vi "transfer char run_subvi_14_2014 05 29_JWb.vi"(0 "VISA session":refnum<visa-resource-name>="GPIB0::17::INSTR", 1 "Y2 axis settings":T6={"Y2 axis on/off"=FALSE, "MINIMUM"=0.0, "MAXIMUM"=1.0, "Variable name"="Ig", "LIN or LOG axis"="LIN"} {"MAXIMUM" format="%.9f"; "MINIMUM" format="%.9f"}, 3 "LKG Path":path, 5 "Var1 sweep settings":T8={"start"=40.0, "stop"=-40.0, "step (linear only)"=-1.0, "sweep spacing (linear: 0)"=0, "sweep mode"=FALSE, "compliance (V)"=100.0, "compliance (A)"=0.001} {"compliance (A)" format="%^.2e"; "compliance (V)" format="%.2f"; "sweep spacing (linear: 0)" items=["linear", "log 10", "log 25", "log 50"]; "step (linear only)" format="%.2f"; "stop" format="%.2f"; "start" format="%.2f"}, 7 "Var2 step settings":T7={"compliance (A)"=0.001, "compliance (V)"=100.0, "start"=-2.0, "total points"=2, "step"=-38.0} {"step" format="%.2f"; "start" format="%.2f"; "compliance (V)" format="%.2f"; "compliance (A)" format="%^.2e"}, 9 "integration time":u32(slide) scale=0.0..2.0, 11 "Input Path":path, 12 "Dielectric Constant":dbl=5.0, 13 "Sample Properties:":T5 {"Date Created" format="%<%x>T"}) -> (2 "Check Cluster":T3, 4 "Output":T4 {"Mobility-Lin" format="%#_4e"; "Mobility-Sat" format="%#_4e"}, 6 "Graph Cluster":T2, 15 "error?":errorcluster)   [LabVIEW 2012]
uses:
  <vilib>/Utility/file.llb/Write To Spreadsheet File (DBL).vi
panel:
  in  "SMU Config":T1={"Vname"="Vs", "Vname 2"="Vd", "Vname 3"="Vg", "Vname 4"="V4", "Iname"="Is", "Iname 2"="Id", "Iname 3"="Ig", "Iname 4"="I4", "Mode"=4, "Mode 2"=0, "Mode 3"=0, "Mode 4"=0, "Function"=4, "Function 2"=2, "Function 3"=1, "Function 4"=4, "Value (V or A)"=0.0, "Value (Either V or A) 2"=0.0, "Value (Either V or A) 3"=0.0, "Value (Either V or A) 4"=0.0} {"Function" items=["disabled", "Var1", "Var2", "Var1'", "Constant"]; "Mode" items=["V", "I", "VPulse", "IPulse", "Common"]; "Function 4" items=["disabled", "Var1", "Var2", "Var1'", "Constant"]; "Mode 4" items=["V", "I", "VPulse", "IPulse", "Common"]; "Function 3" items=["disabled", "Var1", "Var2", "Var1'", "Constant"]; "Mode 3" items=["V", "I", "VPulse", "IPulse", "Common"]; "Function 2" items=["disabled", "Var1", "Var2", "Var1'", "Constant"]; "Mode 2" items=["V", "I", "VPulse", "IPulse", "Common"]}
  in  "Output Path":path
  in  "Temp (K)":dbl=0.001 format="%^.2e"
  in  "NumPts":dbl=5.0
  out "Numeric":dbl
  out "min r":dbl
  out "max r":dbl
  out "error? 2":errorcluster
  in  "MAXIMUM":ext format="%.2e"
  in  "MINIMUM":ext=-1e-05 format="%_2e"
  out "Gate Current Plot":cluster{"trace":dbl[], "trace":dbl[]}(graph)
  in  "Y1 axis":string="Id"
  out "graphic display":cluster{"trace":dbl[], "trace":dbl[]}(graph)
  in  "wait time parameter":dbl=1.0
  in  "compliance (A)":dbl=0.001 format="%^.2e"
  in  "compliance (V)":dbl=100.0 format="%^.2e"
  in  "reset":bool=TRUE
  # "SMU1"
  # "SMU2"
  # "SMU3"
  # "SMU4"
  # "Sample Properties:"
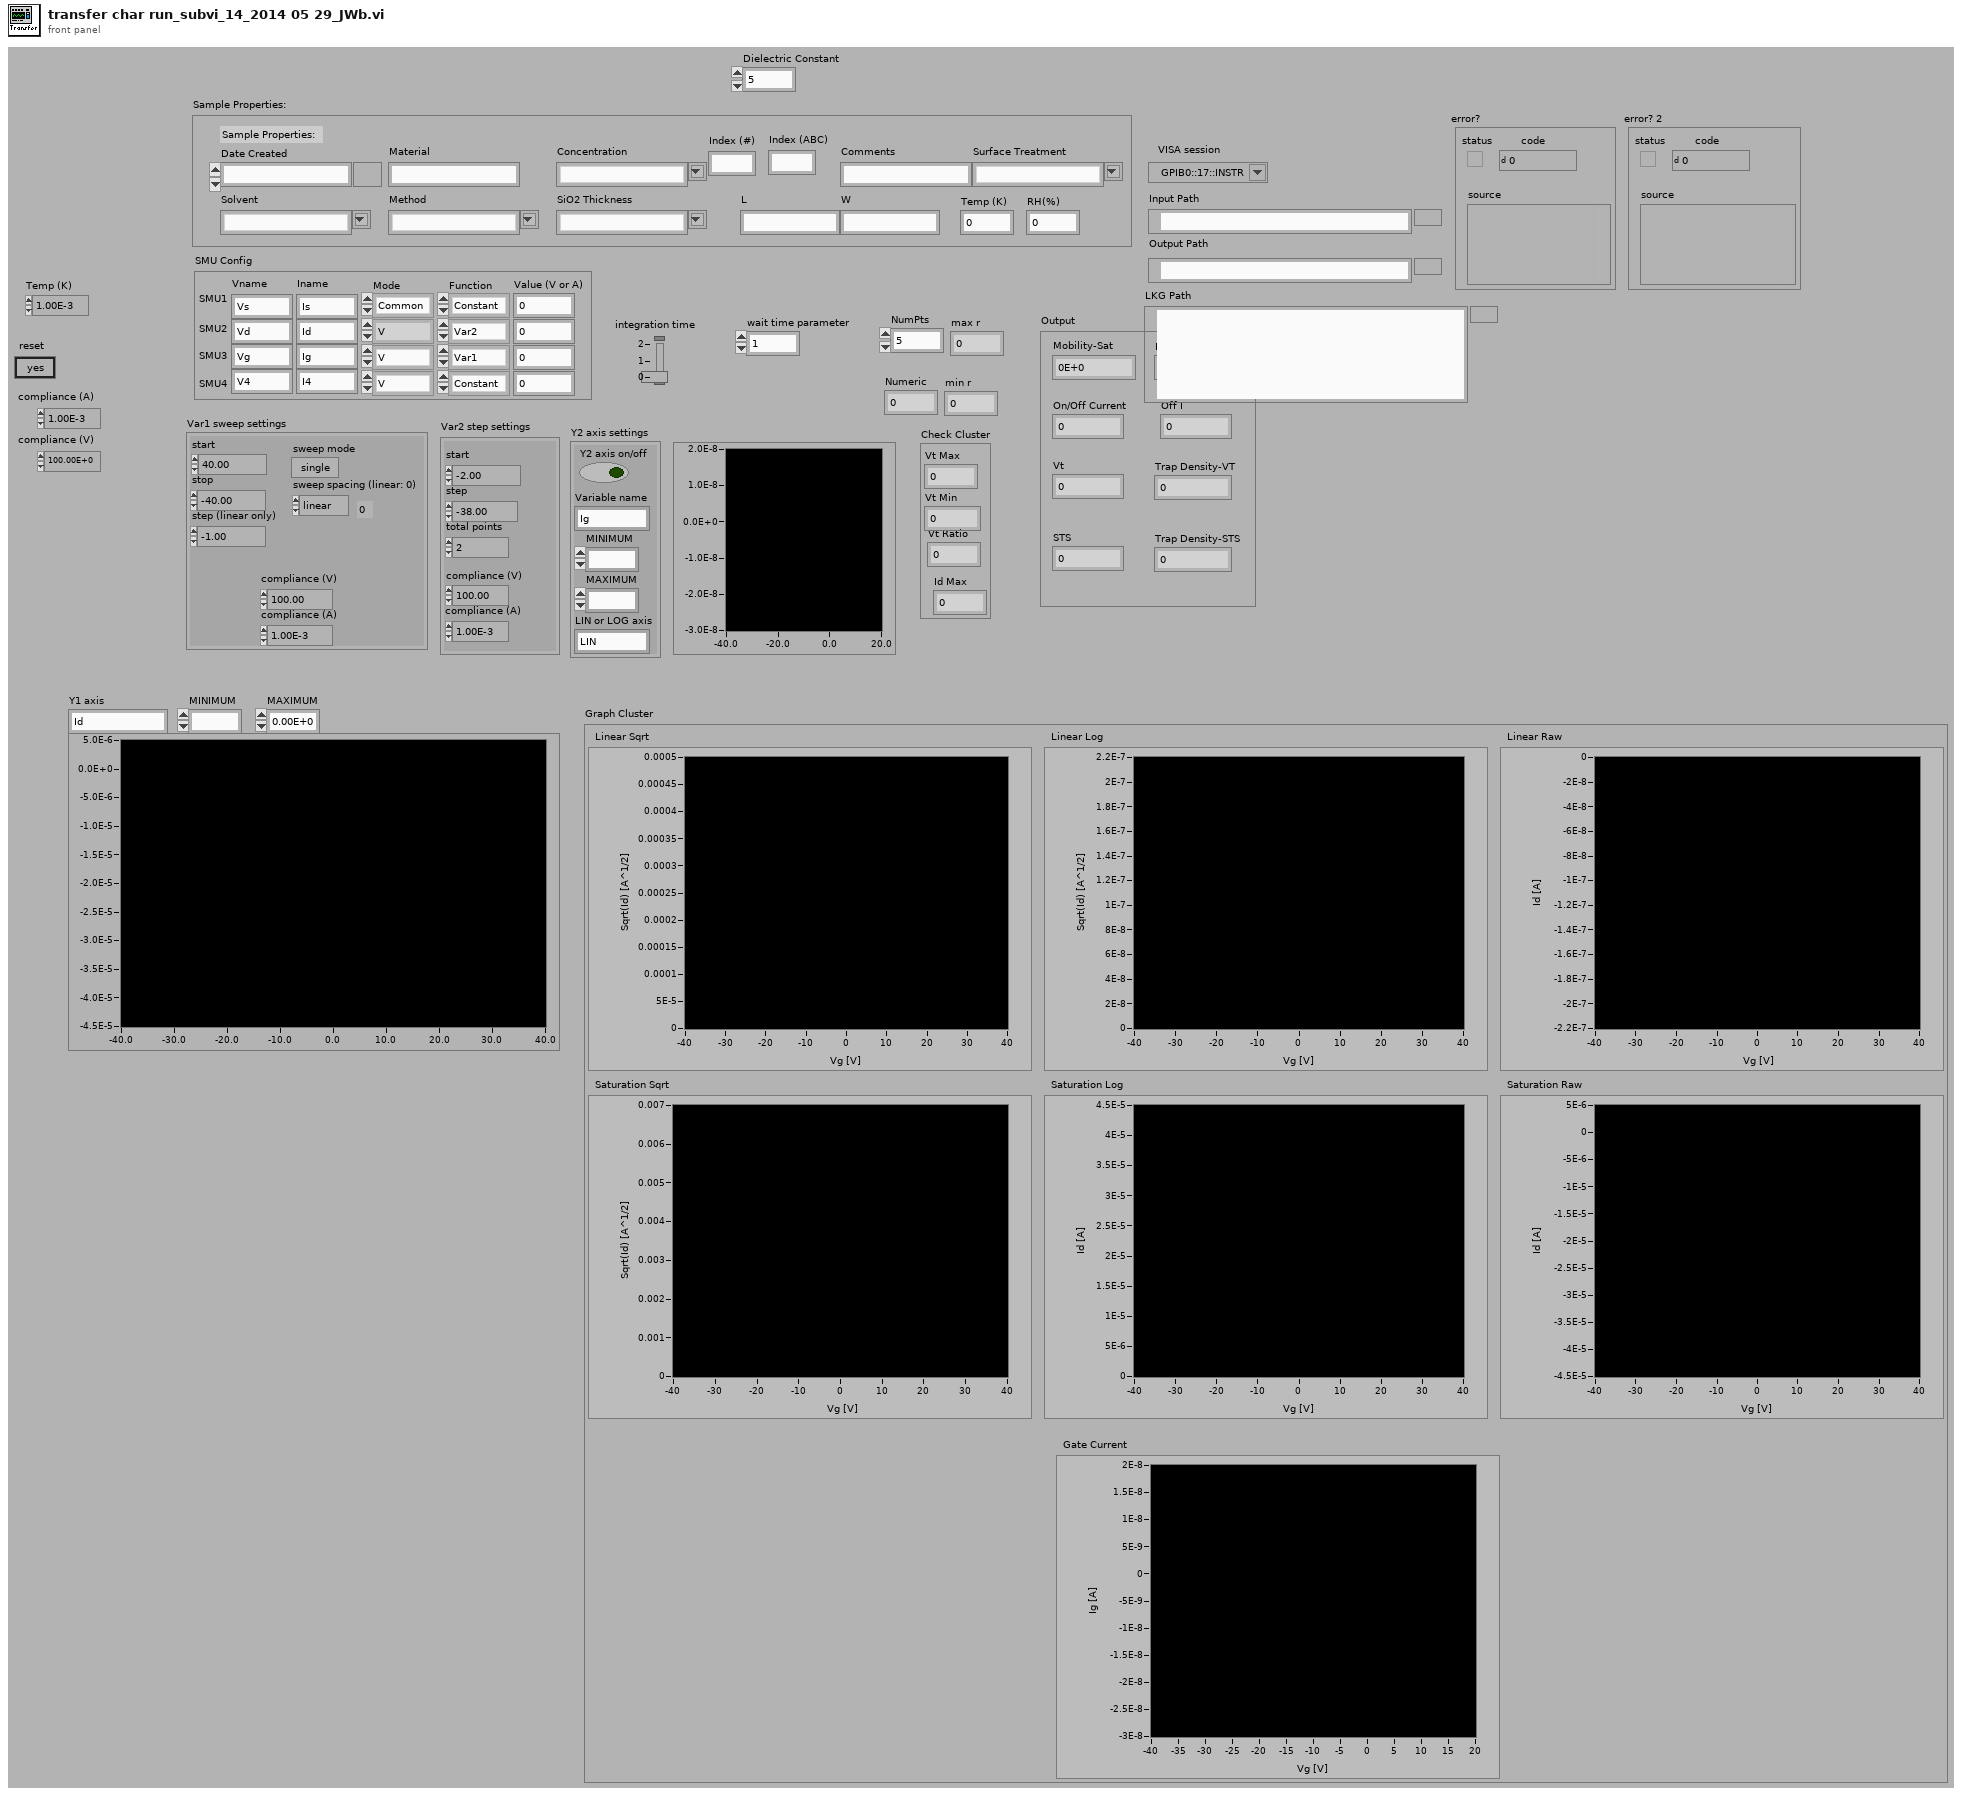
[diagram p1: front panel]
types:
  T1 = cluster{"Vname":string, "Vname 2":string, "Vname 3":string, "Vname 4":string, "Iname":string, "Iname 2":string, "Iname 3":string, "Iname 4":string, "Mode":u16, "Mode 2":u16, "Mode 3":u16, "Mode 4":u16, "Function":u16, "Function 2":u16, "Function 3":u16, "Function 4":u16, "Value (V or A)":dbl, "Value (Either V or A) 2":dbl, "Value (Either V or A) 3":dbl, "Value (Either V or A) 4":dbl}
  T2 = cluster{"Linear Sqrt":cluster{dbl[], "trace":dbl[]}[], "Linear Log":cluster{dbl[], "trace":dbl[]}[], "Linear Raw":cluster{dbl[], dbl[]}[], "Saturation Sqrt":cluster{dbl[], "trace":dbl[]}[], "Saturation Log":cluster{dbl[], "trace":dbl[]}[], "Saturation Raw":cluster{dbl[], "trace":dbl[]}[], "Gate Current":cluster{dbl[], "trace":dbl[]}[]}
  T3 = cluster{"Vt Max":i32, "Vt Min":i32, "Vt Ratio":i32, "Id Max":dbl}
  T4 = cluster{"Mobility-Sat":dbl, "Mobility-Lin":dbl, "On/Off Current":dbl, "Off I":dbl, "Vt":dbl, "STS":dbl, "Trap Density-VT":dbl, "Trap Density-STS":dbl}
  T5 = cluster{"Date Created":timestamp, "Material":string, "Solvent":string, "Concentration":string, "Method":string, "SiO2 Thickness":string, "Index (#)":string, "Index (ABC)":string, "L":string, "W":string, "Surface Treatment":string, "Comments":string, "Temp (K)":dbl, "RH(%)":dbl}
  T6 = cluster{"Y2 axis on/off":bool, "MINIMUM":ext, "MAXIMUM":ext, "Variable name":string, "LIN or LOG axis":string}
  T7 = cluster{"compliance (A)":dbl, "compliance (V)":dbl, "start":dbl, "total points":u16, "step":dbl}
  T8 = cluster{"start":dbl, "stop":dbl, "step (linear only)":dbl, "sweep spacing (linear: 0)":u16, "sweep mode":bool, "compliance (V)":dbl, "compliance (A)":dbl}
  T9 = cluster{"Vt Max":dbl, "Vt Min":dbl, "Vt Ratio":dbl, "Id Max":dbl}
  T10 = cluster{"Mobility-Sat":dbl, "Mobility-Lin":dbl, "On/Off I-Sat":dbl, "Off I-Sat":dbl, "VT-Sat":dbl, "Sub Threshold Swing":dbl, "Trap Density-VT":dbl, "Trap Density (N)":dbl}
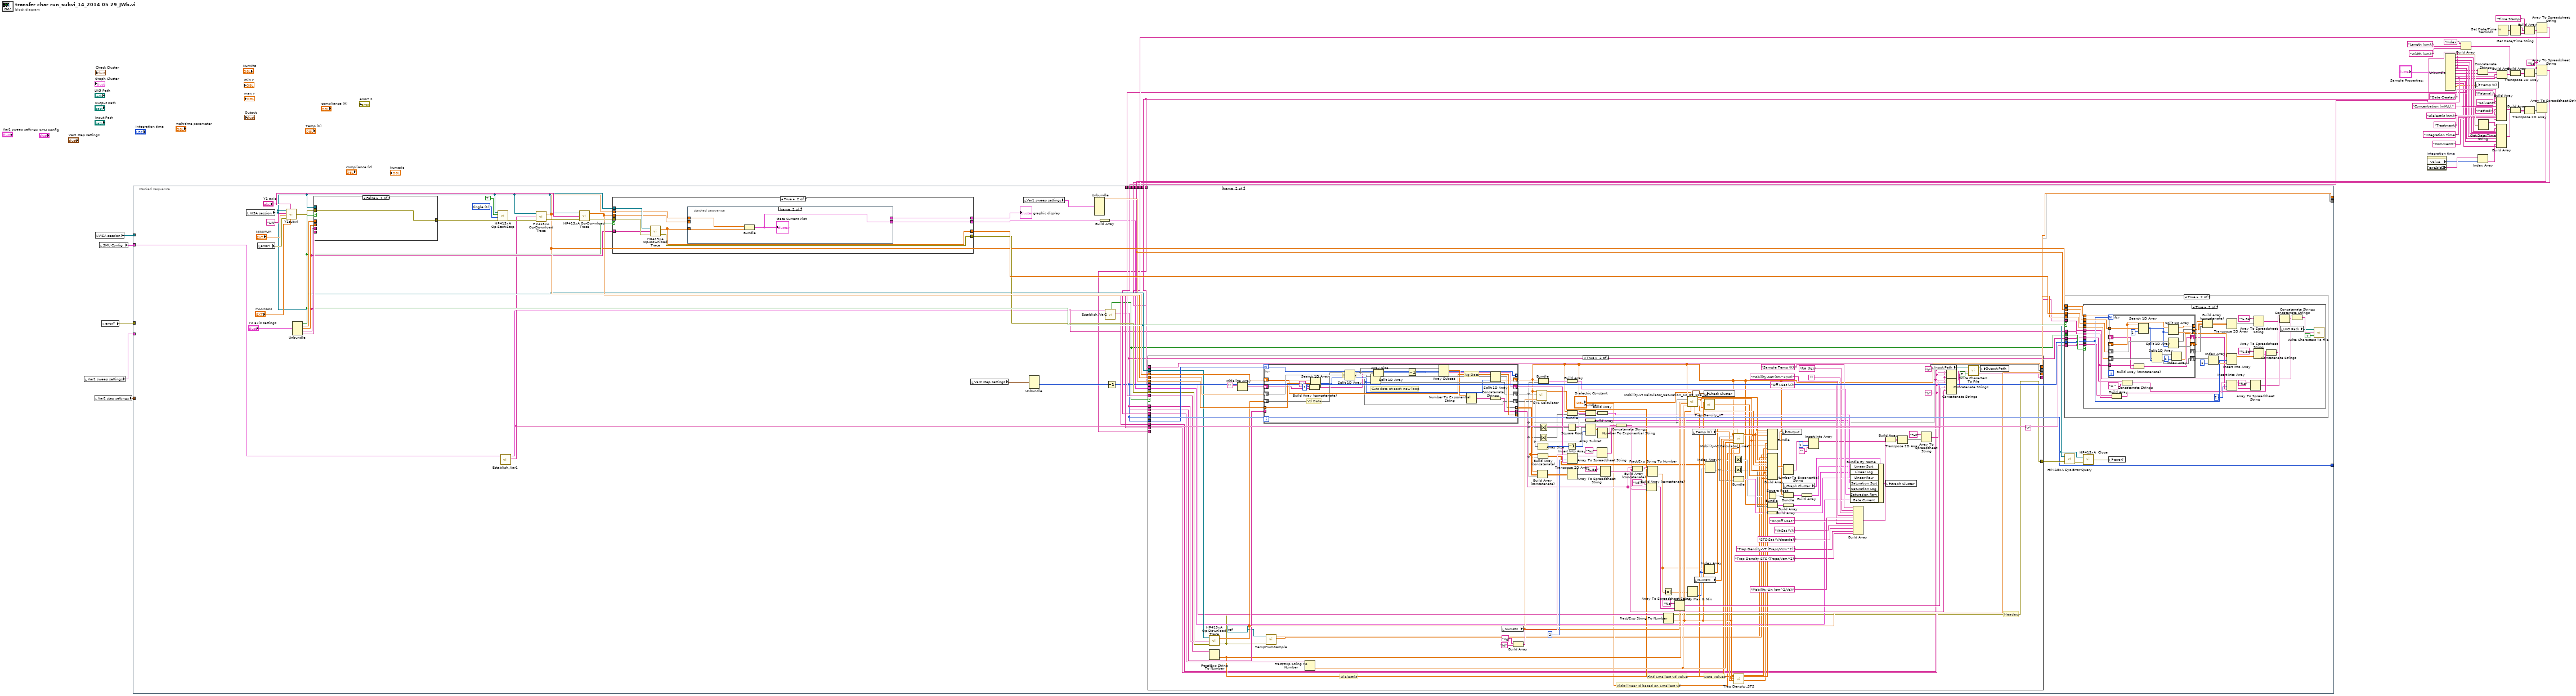
[diagram p0: block diagram]
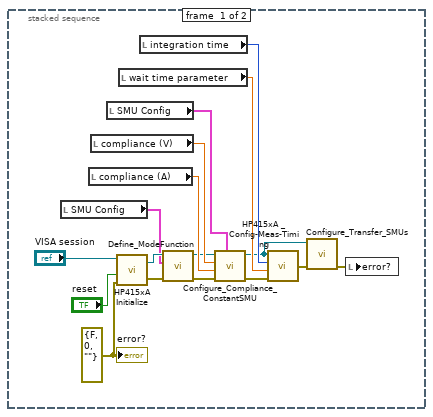
[diagram p2: hidden frame]
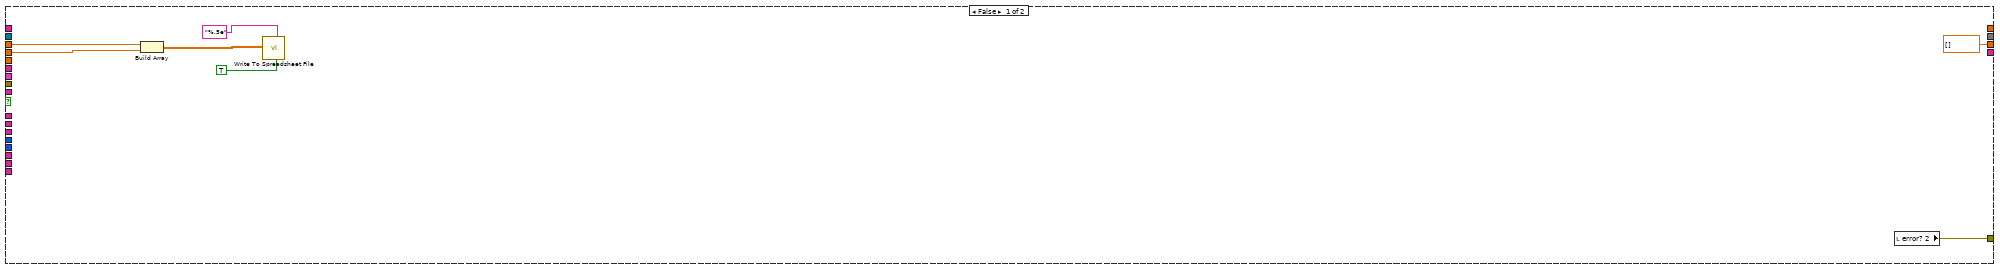
[diagram p3: hidden frame]
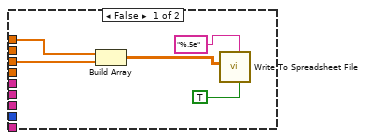
[diagram p5: hidden frame]
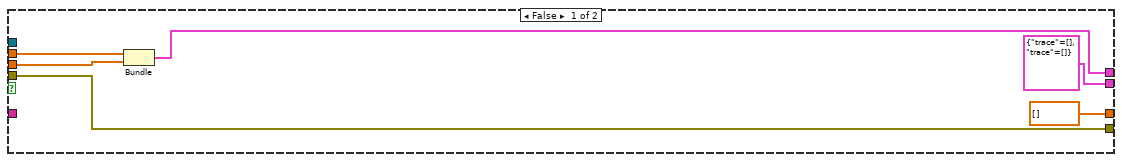
[diagram p6: hidden frame]
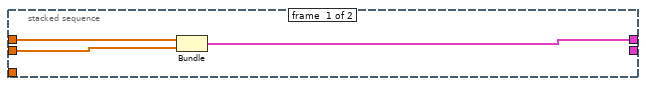
[diagram p7: hidden frame]
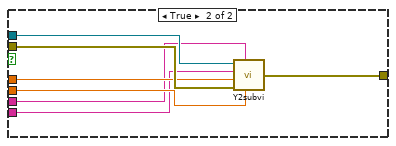
[diagram p8: hidden frame]
diagram:
  w12 = "%s"
  n1 = local read "Var1 sweep settings"() -> (w4:T8)
  n2 = local read "Var2 step settings"() -> (w3:T7)
  n3 = local read "VISA session"() -> (w2:refnum<visa-resource-name>)
  n4 = local read "SMU Config"() -> (w5:T1)
  n5 = local read "error?"() -> (w1:errorcluster)
  n6 = property on="integration time" class="Slide (strict)"() -> ("Value"=w7:u32, "TextLbls[]"=w8:string[])  [unwired: 2 in, 2 out]
  n7 = Unbundle("Sample Properties:") -> ("Date Created"=w26:timestamp, "Material"=w25:string, "Solvent"=w22:string, "Concentration"=w21:string, "Method"=w24:string, "SiO2 Thickness"=w13:string, "Index (#)"=w17:string, "Index (ABC)"=w16:string, "L"=w19:string, "W"=w20:string, "Surface Treatment"=w18:string, "Comments"=w9:string, "Temp (K)"=w14:dbl)  [unwired: 1 out]
  n8 = Build Array("Index:", "Length (um):", "Width (um):") -> (w32:string[])
  n9 = local write "Temp (K)"(w14) -> ()
  n10 = Concatenate Strings(w17, w16) -> (w15:string)
  n11 = Index Array(array=w8, index=w7) -> (element=w6:string)
  n12 = Get Date/Time String(seconds (now)=w26) -> (date string=w52:string)  [unwired: 2 in, 1 out]
  n13 = Build Array("Date Created:", "Material:", "Solvent:", "Concentration (mM/L):", "Method:", "Dielectric (nm):", "Treatment:", "Integration Time:", "Comments:") -> (w36:string[])
  n14 = Build Array(w52, w25, w22, w21, w24, w13, w18, w6, w9) -> (w35:string[])
  n15 = Build Array(w15, w19, w20) -> (w31:string[])
  n16 = Get Date/Time In Seconds() -> (seconds since 1Jan1904=w47:timestamp)
  n17 = Get Date/Time String(seconds (now)=w47) -> (date string=w46:string, time string=w45:string)  [unwired: 2 in]
  n18 = Build Array(w32, w31) -> (w30:string[][])
  n19 = Build Array(w36, w35) -> (w34:string[][])
  n20 = Build Array("Time Stamp:", w46, w45) -> (w44:string[])
  n21 = Transpose 2D Array(2D array=w30) -> (transposed array=w29:string[][])
  n22 = Transpose 2D Array(2D array=w34) -> (transposed array=w33:string[][])
  n23 = Array To Spreadsheet String(array=w44, 3:w12) -> (spreadsheet string=w37:string)  [unwired: 1 in]
  n24 = Array To Spreadsheet String(array=w29, 3:w12) -> (spreadsheet string=w28:string)  [unwired: 1 in]
  n25 = Array To Spreadsheet String(array=w33, 3:w12) -> (spreadsheet string=w40:string)  [unwired: 1 in]
  n26 = stacked-sequence {
    tunnel: w37 -> [_ w90]
    tunnel: w40 -> [_ w89]
    tunnel: w28 -> [_ w88]
    tunnel: [_ w87] -> _
    tunnel: [_ w86] -> _
    tunnel: [_ w83] -> _
    tunnel: w20 -> [_ w85]
    tunnel: w19 -> [_ w84]
    tunnel: w13 -> [_ w82]
    tunnel: w13 -> [_ w81]
    tunnel: w5 -> [_ w73]
    tunnel: w4 -> [_ _]
    tunnel: w3 -> [_ _]
    tunnel: w2 -> [_ _]
    tunnel: w1 -> [_ _]
    frame #0 {
      w69 = errorcluster {"status"=FALSE, "code"=0, "source"=""} ("error out")
      n27 = local read "SMU Config"() -> (w64:T1)
      n28 = local read "compliance (A)"() -> (w65:dbl)
      n29 = local read "compliance (V)"() -> (w66:dbl)
      n30 = local read "SMU Config"() -> (w63:T1)
      n31 = call "HP415xA  Initialize.vi"("instrument descriptor"="VISA session", "reset"="reset", "error in (no error)"=w69) -> ("VISA session"=w67:refnum<visa-resource-name>, "error out"=w58:errorcluster)  [unwired: 2 in]
      n32 = local read "wait time parameter"() -> (w60:dbl)
      n33 = local read "integration time"() -> (w59:u32)
      n34 = call "Define_ModeFunction.vi"("error in (no error)"=w58, "SMU Config"=w64, "VISA Refnum in"=w67) -> ("error out"=w57:errorcluster, "VISA Refnum out"=w55:refnum<visa-resource-name>)  [unwired: 7 in]
      n35 = call "Configure_Compliance_ConstantSMU.vi"("SMU Config"=w63, "error in (no error)"=w57, "compliance (A)"=w65, "compliance (V)"=w66, "VISA In"=w55) -> ("error out"=w56:errorcluster, "VISA Out"=w54:refnum<visa-resource-name>)  [unwired: 5 in]
      n36 = call "HP415xA _Config-Meas-Timing.vi"("error in (no error)"=w56, "wait time parameter"=w60, "integration time"=w59, "VISA session"=w54) -> ("error out"=w61:errorcluster)  [unwired: 2 in]
      n37 = call "Configure_Transfer_SMUs.vi"("error in (no error)"=w61, "VISA In"=w54) -> ("error out"=w62:errorcluster)  [unwired: 8 in, 1 out]
      n38 = local write "error?"(w62) -> ()
      "error?" <- w69
    }
    frame #1 {
      w113 = u32 1 items=["stop  ", "single  ", "single-append  ", "stress start  ", "continuous  ", "standby on  ", "standby off  ", "zero  "] ("function (stop:0)")
      n39 = local read "VISA session"() -> (w92:refnum<visa-resource-name>)
      n40 = local read "error?"() -> (w105:errorcluster)
      n41 = call "Y1subvi.vi"("MAXIMUM"="MAXIMUM", "Variable name"="Y1 axis", "error in (no error)"=w105, "MINIMUM"="MINIMUM", "LIN or LOG axis"="LIN", "VISA resource name"=w92) -> ("error out"=w106:errorcluster)
      n42 = Unbundle("Y2 axis settings") -> ("Y2 axis on/off"=w99:bool, "MINIMUM"=w110:ext, "MAXIMUM"=w109:ext, "Variable name"=w76:string, "LIN or LOG axis"=w108:string)
      n43 = case shown="False" w99 {
        tunnel: w106 -> [w358 w365]
        tunnel: w92 -> [_ w364]
        tunnel: w110 -> [_ w363]
        tunnel: w109 -> [_ w362]
        tunnel: w76 -> [_ w361]
        tunnel: w108 -> [_ w360]
        tunnel: [w358 w359] -> w107
        frame False {
        }
        frame True {
          n44 = call "Y2subvi.vi"("MAXIMUM"=w362, "Variable name"=w361, "error in (no error)"=w365, "MINIMUM"=w363, "LIN or LOG axis"=w360, "VISA resource name"=w364) -> ("error out"=w359:errorcluster)
        }
      }
      n45 = call "HP415xA Op-Start-Stop.vi"("error in (no error)"=w107, "function (stop:0)"=w113, "wait until finish"=TRUE, "VISA session"=w92) -> ("error out"=w112:errorcluster)  [unwired: 6 in, 1 out]
      n46 = call "Establish_Var1.vi"("SMU Config In"=w73) -> ("Vname"=w75:string, "SMU Config Out"=w71:T1)  [unwired: 8 in]
      n47 = call "HP415xA Op-Download Trace.vi"("error in (no error)"=w112, "trace (variable) name"=w75, "VISA session"=w92) -> ("error out"=w120:errorcluster, "trace"=w97:dbl[])
      n48 = call "HP415xA Op-Download Trace.vi"("error in (no error)"=w120, "trace (variable) name"="Y1 axis", "VISA session"=w92) -> ("error out"=w102:errorcluster, "trace"=w93:dbl[])
      n49 = case shown="True" w99 {
        tunnel: w102 -> [w342 w351]
        tunnel: w92 -> [_ w350]
        tunnel: w76 -> [_ w349]
        tunnel: [w342 w348] -> w94
        tunnel: w97 -> [w340 w347]
        tunnel: w93 -> [w341 w346]
        tunnel: [w339 w345] -> w79
        tunnel: [dbl[] [] ("trace") w344] -> w98
        tunnel: [cluster{"trace":dbl[], "trace":dbl[]} {"trace"=[], "trace"=[]} w343] -> w77
        frame False {
          n50 = Bundle("trace"=w340, "trace"=w341) -> (w339:cluster{"trace":dbl[], "trace":dbl[]})  [unwired: 1 in]
        }
        frame True {
          n51 = call "HP415xA Op-Download Trace.vi"("error in (no error)"=w351, "trace (variable) name"=w349, "VISA session"=w350) -> ("error out"=w348:errorcluster, "trace"=w344:dbl[])
          n52 = stacked-sequence {
            tunnel: w344 -> [_ w357]
            tunnel: w347 -> [w354 w356]
            tunnel: w346 -> [w353 _]
            tunnel: [w352 _] -> w345
            tunnel: [_ w355] -> w343
            frame #0 {
              n53 = Bundle("trace"=w354, "trace"=w353) -> (w352:cluster{"trace":dbl[], "trace":dbl[]})  [unwired: 1 in]
            }
            frame #1 {
              n54 = Bundle("trace"=w356, "trace"=w357) -> (w355:cluster{"trace":dbl[], "trace":dbl[]})  [unwired: 1 in]
              "Gate Current Plot" <- w355
            }
          }
        }
      }
      "graphic display" <- w79
      n55 = local read "Var2 step settings"() -> (w116:T7)
      n56 = local read "Var1 sweep settings"() -> (w117:T8)
      n57 = Unbundle(w116) -> ("total points"=w115:u16)  [unwired: 4 out]
      n58 = Unbundle(w117) -> ("start"=w91:dbl)  [unwired: 6 out]
      n59 = Build Array(w77) -> (w78:cluster{"trace":dbl[], "trace":dbl[]}[])
      n60 = call "Establish_Var2.vi"("SMU Config In"=w71) -> ("Vname"=w80:string, "Execute?"=w72:bool)  [unwired: 8 in, 1 out]
      n61 = Decrement(x=w115) -> (x-1=w83:u16)
      n62 = case shown="True" w72 {
        tunnel: w91 -> [_ w247]
        tunnel: w93 -> [w125 w246]
        tunnel: w97 -> [w126 w245]
        tunnel: w83 -> [_ w244]
        tunnel: w92 -> [_ w240]
        tunnel: w94 -> [_ w239]
        tunnel: [w127 w131] -> w96
        tunnel: w80 -> [_ w238]
        tunnel: w80 -> [_ w233]
        tunnel: [dbl[] [] ("trace") w237] -> w95
        tunnel: w90 -> [_ w141]
        tunnel: w89 -> [_ w139]
        tunnel: w88 -> [_ w138]
        tunnel: [_ w150] -> w87
        tunnel: [_ w145] -> w86
        tunnel: w85 -> [_ w216]
        tunnel: w84 -> [_ w215]
        tunnel: w83 -> [_ _]
        tunnel: w82 -> [_ _]
        tunnel: w81 -> [_ w199]
        tunnel: w78 -> [_ w142]
        tunnel: [_ w134] -> w74
        frame False {
          n63 = Build Array(w126, w125) -> (w122:dbl[][])
          n64 = call-poly <vilib>:"Write To Spreadsheet File.vi"("transpose? (no:F)"=TRUE ("append to file? (new file:F)"), "format (%.3f)"="%.5e", "2D data"=w122) -> ()  [unwired: 5 in, 1 out]
          n65 = local read "error? 2"() -> (w127:errorcluster)
        }
        frame True {
          (unwired) "\r"
          w137 = "\r"
          w140 = "\r"
          # "Find Smallest Vd Value"
          # "Picks linear Id based on Smallest Vd"
          # "Dielectric"
          # "Data Values"
          # "Headers"
          n66 = call "HP415xA Op-Download Trace.vi"("error in (no error)"=w239, "trace (variable) name"=w238, "VISA session"=w240) -> ("error out"=w131:errorcluster, "trace"=w237:dbl[])
          n67 = Fract/Exp String To Number(string=w215) -> (number=w197:dbl)  [unwired: 3 in, 1 out]
          n68 = Initialize Array("") -> (w217:string[])  [unwired: 1 in]
          n69 = for {
            N: w244 -> [w248]
            shift-right: [w265] -> w150
            shift-left: w245 -> [w261]
            tunnel: w247 -> [w267]
            tunnel: [w266] -> _ mode=indexing
            shift-right: [w262] -> w145
            shift-left: w246 -> [w264]
            tunnel: [w263] -> w193 mode=indexing
            shift-right: [w258] -> w136
            shift-left: w237 -> [w260]
            tunnel: w233 -> [_]
            tunnel: [w252] -> w194 mode=indexing
            shift-right: [w251] -> w221
            shift-left: w217 -> [w250]
            tunnel: [w248] -> _ mode=indexing
            # "Cuts data at each new loop"
            # "Id Data"
            # "Vd Data"
            # "Vg Data"
            n70 = Build Array (concatenate)("Id", w250) -> (w251:string[])
            n71 = Search 1D Array(1D array=w261, element=w267, start index (0)=1) -> (index of element=w259:i32)
            n72 = Split 1D Array(array=w260, index=w259) -> (first subarray=w256:dbl[], second subarray=w258:dbl[])
            n73 = Split 1D Array(array=w264, index=w259) -> (first subarray=w263:dbl[], second subarray=w262:dbl[])
            n74 = Array Size(array=w256) -> (size(s)=w255:i32)
            n75 = Decrement(x=w255) -> (x-1=w254:i32)
            n76 = Array Subset(array=w256, index=w254) -> (w257:dbl[])  [unwired: 1 in]
            n77 = Number To Exponential String(number=w257) -> (E-format string=w253:string[])  [unwired: 3 in]
            n78 = Split 1D Array(array=w261, index=w259) -> (first subarray=w266:dbl[], second subarray=w265:dbl[])
            n79 = Concatenate Strings(w253) -> (w252:string)
          }
          n80 = call "TempHumSample.vi"("VISA resource name"=refnum<visa-resource-name> "COM4", "error in (no error)"=w131) -> ("CurHum"=w129:dbl, "CurTemp"=w128:dbl)  [unwired: 6 in, 1 out]
          n81 = Fract/Exp String To Number(string=w216) -> (number=w198:dbl)  [unwired: 3 in, 1 out]
          n82 = local read "NumPts"() -> (w190:dbl)
          n83 = Build Array("Vg", "Id") -> (w222:string[])
          n84 = call "STS Calculator.vi"("NumPts"=w190, "Saturation Id"=w145, "Vg Column"=w150) -> ("Sub Threshold Swing"=w183:dbl)  [unwired: 5 in, 3 out]
          n85 = Build Array (concatenate)(w150, w193, w145) -> (w243:dbl[][])
          n86 = Array Size(array=w136) -> (size(s)=w231:i32)
          n87 = Build Array (concatenate)(w193, w145) -> (w175:dbl[][])
          n88 = Bundle("trace"=w150, "trace"=w145) -> (w163:cluster{"trace":dbl[], "trace":dbl[]})  [unwired: 1 in]
          n89 = Absolute Value(x=w145) -> (abs(x)=w149:dbl[])
          n90 = Absolute Value(x=w145) -> (abs(x)=w144:dbl[])
          n91 = Square Root(x=w149) -> (sqrt(x)=w148:dbl[])
          n92 = Decrement(x=w231) -> (x-1=w230:i32)
          n93 = Build Array(w163) -> (w162:cluster{"trace":dbl[], "trace":dbl[]}[])
          n94 = Bundle("trace"=w150, w144) -> (w158:cluster{"trace":dbl[], dbl[]})  [unwired: 1 in]
          n95 = Insert Into Array(array=w222, index=2, new element=w221) -> (w220:string[])
          n96 = Transpose 2D Array(2D array=w243) -> (transposed array=w241:dbl[][])
          n97 = Bundle("trace"=w150, w148) -> (w159:cluster{"trace":dbl[], dbl[]})  [unwired: 1 in]
          n98 = Build Array(w158) -> (w157:cluster{"trace":dbl[], dbl[]}[])
          n99 = Array Subset(array=w136, index=w230) -> (w229:dbl[])  [unwired: 1 in]
          n100 = Array To Spreadsheet String(array=w220, 3:"%s") -> (spreadsheet string=w226:string)  [unwired: 1 in]
          n101 = Build Array(w159) -> (w156:cluster{"trace":dbl[], dbl[]}[])
          n102 = Number To Exponential String(number=w229) -> (E-format string=w225:string[])  [unwired: 3 in]
          n103 = Array To Spreadsheet String(array=w241, 3:"%.5e" ("format string")) -> (spreadsheet string=w234:string)  [unwired: 1 in]
          n104 = Concatenate Strings(w225) -> (w135:string)
          n105 = Build Array (concatenate)(w194, w135) -> (w192:string[])
          n106 = Build Array (concatenate)("Vd=", w194, w135) -> (w228:string[])
          n107 = Fract/Exp String To Number(string=w192) -> (number=w177:dbl[])  [unwired: 3 in, 1 out]
          n108 = Absolute Value(x=w177) -> (abs(x)=w178:dbl[])
          n109 = Fract/Exp String To Number(string=w199) -> (number=w191:dbl)  [unwired: 3 in, 1 out]
          n110 = Array To Spreadsheet String(array=w228, 3:"%s") -> (spreadsheet string=w232:string)  [unwired: 1 in]
          n111 = call "Mobility-Vt Calculator_Saturation_12_09_10a_JW.vi"("Vg Column"=w150, "Dielectric Constant"="Dielectric Constant", "Sat Id Column"=w145, "NumPts"=w190, "Length"=w197, "Width"=w198, "Dielectric Thickness"=w191) -> ("Check Cluster"=w179:T9, "Mobility-Sat"=w188:dbl, "VT-Sat"=w184:dbl, "Off I-Sat"=w185:dbl, "On/Off I-Sat"=w186:dbl)  [unwired: 4 out]
          n112 = Array Max & Min(array=w178) -> (min index (indices)=w174:i32)  [unwired: 3 out]
          n113 = local read "Temp (K)"() -> (w189:dbl)
          n114 = local read "NumPts"() -> (w196:dbl)
          n115 = local write "Check Cluster"(w179) -> ()
          n116 = call "Trap Density_VT.vi"("VT"=w184, "Dielectric"=w191) -> ("Trap Density-VT"=w182:dbl)
          n117 = Index Array(array=w177, index=w174) -> (element=w176:dbl)
          n118 = Index Array(array=w175, index (row)=w174) -> (element=w147:dbl[])  [unwired: 1 in]
          n119 = Absolute Value(x=w147) -> (abs(x)=w152:dbl[])
          n120 = Absolute Value(x=w147) -> (abs(x)=w146:dbl[])
          n121 = call "Mobility-Vt Calculator_Linear.vi"("Vg Column"=w150, "Vd"=w176, "Lin Id Column"=w147, "NumPts"=w196, "Length"=w197, "Width"=w198, "Dielectric Thickness"=w191, "Dielectric Constant"="Dielectric Constant") -> ("Mobility-Lin"=w187:dbl)  [unwired: 1 in, 6 out]
          n122 = Bundle("trace"=w150, w147) -> (w161:cluster{"trace":dbl[], dbl[]})  [unwired: 1 in]
          n123 = call "Trap Density_STS.vi"("Temp (T) [K]"=w189, "S.T.S. (S)"=w183, "Dielectric"=w191) -> ("Trap Density (N)"=w181:dbl)  [unwired: 8 in]
          n124 = Square Root(x=w152) -> (sqrt(x)=w151:dbl[])
          n125 = Bundle("Mobility-Sat"=w188, "Mobility-Lin"=w187, "On/Off I-Sat"=w186, "Off I-Sat"=w185, "VT-Sat"=w184, "Sub Threshold Swing"=w183, "Trap Density-VT"=w182, "Trap Density (N)"=w181) -> (w180:T10)  [unwired: 1 in]
          n126 = Build Array(w128, w129, w188, w187, w186, w185, w184, w183, w182, w181) -> (w212:dbl[])
          n127 = Bundle("trace"=w150, w146) -> (w155:cluster{"trace":dbl[], dbl[]})  [unwired: 1 in]
          n128 = Build Array(w161) -> (w160:cluster{"trace":dbl[], dbl[]}[])
          n129 = local write "Output"(w180) -> ()
          n130 = Number To Exponential String(number=w212) -> (E-format string=w172:string[])  [unwired: 3 in]
          n131 = local read "Graph Cluster"() -> (w165:T2)
          n132 = Bundle("trace"=w150, w151) -> (w154:cluster{"trace":dbl[], dbl[]})  [unwired: 1 in]
          n133 = Build Array(w155) -> (w143:cluster{"trace":dbl[], dbl[]}[])
          n134 = Build Array(w154) -> (w153:cluster{"trace":dbl[], dbl[]}[])
          n135 = Insert Into Array(array=w172, index=1, new element="") -> (w169:string[])
          n136 = Bundle By Name(cluster=w165, "Linear Sqrt"=w153, "Linear Log"=w143, "Linear Raw"=w160, "Saturation Sqrt"=w156, "Saturation Log"=w157, "Saturation Raw"=w162, "Gate Current"=w142) -> (w164:T2)
          n137 = Build Array("Sample Temp (K):", "RH (%):", "", "Mobility-Sat (cm^2/Vs):", "Mobility-Lin (cm^2/Vs):", "On/Off I-Sat:", "Off I-Sat (A):", "Vt-Sat (V):", "STS-Sat (V/decade):", "Trap Density-VT (Traps/Vcm^2):", "Trap Density-STS (Traps/Vcm^2):") -> (w213:string[])
          n138 = Build Array(w213, w169) -> (w168:string[][])
          n139 = local write "Graph Cluster"(w164) -> ()
          n140 = Transpose 2D Array(2D array=w168) -> (transposed array=w167:string[][])
          n141 = Array To Spreadsheet String(array=w167, 3:"%s") -> (spreadsheet string=w210:string)  [unwired: 1 in]
          n142 = local read "Input Path"() -> (w200:path)
          n143 = Concatenate Strings(w141, w140, w139, w140, w138, w210, w140, w232, w226, w234, w137) -> (w236:string)
          n144 = Concatenate Strings(w141, w140, w139, w137, w138, w137) -> (w134:string)
          n145 = call <vilib>:"Write Characters To File.vi"("append to file? (new file:F)"=TRUE, "character string"=w236, "file path (dialog if empty)"=w200) -> ("new file path (Not A Path if cancelled)"=w208:path)  [unwired: 2 in]
          n146 = local write "Output Path"(w208) -> ()
        }
      }
      n147 = case shown="True" w99 {
        tunnel: w83 -> [_ w277]
        tunnel: w72 -> [_ w278]
        tunnel: w97 -> [_ w276]
        tunnel: w91 -> [_ w275]
        tunnel: w98 -> [_ w274]
        tunnel: w95 -> [_ w273]
        tunnel: w80 -> [_ w272]
        tunnel: w76 -> [_ w271]
        tunnel: w75 -> [_ w270]
        tunnel: w74 -> [_ w269]
        frame False {
        }
        frame True {
          n148 = case shown="True" w278 {
            tunnel: w277 -> [_ w307]
            tunnel: w276 -> [w282 w319]
            tunnel: w275 -> [_ w318]
            tunnel: w274 -> [w283 w317]
            tunnel: w273 -> [_ w316]
            tunnel: w272 -> [_ w304]
            tunnel: w271 -> [_ w297]
            tunnel: w270 -> [_ w296]
            tunnel: w269 -> [_ w285]
            frame False {
              n149 = Build Array(w282, w283) -> (w281:dbl[][])
              n150 = call-poly <vilib>:"Write To Spreadsheet File.vi"("transpose? (no:F)"=TRUE, "format (%.3f)"="%.5e", "2D data"=w281) -> ()  [unwired: 5 in, 1 out]
            }
            frame True {
              n151 = for {
                N: w307 -> [_]
                shift-right: [w333] -> w315
                shift-left: w319 -> [w334]
                tunnel: w318 -> [w336]
                tunnel: [w332] -> _ mode=indexing
                shift-right: [w329] -> w299
                shift-left: w317 -> [w331]
                tunnel: [w330] -> w314 mode=indexing
                shift-right: [w326] -> w311
                shift-left: w316 -> [w327]
                tunnel: [w323] -> w308 mode=indexing
                shift-right: [w322] -> w298
                shift-left: _ -> [w321]
                tunnel: w297 -> [w320]
                n152 = Build Array (concatenate)(w320, w321) -> (w322:string[])
                n153 = Search 1D Array(1D array=w334, element=w336, start index (0)=1) -> (index of element=w328:i32)
                n154 = Split 1D Array(array=w327, index=w328) -> (first subarray=w324:dbl[], second subarray=w326:dbl[])
                n155 = Split 1D Array(array=w334, index=w328) -> (first subarray=w332:dbl[], second subarray=w333:dbl[])
                n156 = Split 1D Array(array=w331, index=w328) -> (first subarray=w330:dbl[], second subarray=w329:dbl[])
                n157 = Index Array(array=w324, index=1) -> (element=w323:dbl)
              }
              n158 = Build Array(w296, w297) -> (w301:string[])
              n159 = Concatenate Strings(w304, "= " ("string")) -> (w294:string)
              n160 = Build Array (concatenate)(w315, w314, w299) -> (w313:dbl[][])
              n161 = Index Array(array=w311, index=1) -> (element=w309:dbl)
              n162 = Transpose 2D Array(2D array=w313) -> (transposed array=w312:dbl[][])
              n163 = Insert Into Array(array=w308, index=w307, new element=w309) -> (w306:dbl[])
              n164 = Insert Into Array(array=w301, index=2, new element=w298) -> (w300:string[])
              n165 = Array To Spreadsheet String(array=w300, 3:"%s") -> (spreadsheet string=w290:string)  [unwired: 1 in]
              n166 = Array To Spreadsheet String(array=w312, 3:"%.5e" ("format string")) -> (spreadsheet string=w291:string)  [unwired: 1 in]
              n167 = Array To Spreadsheet String(array=w306, 3:"%.5e" ("format string")) -> (spreadsheet string=w293:string)  [unwired: 1 in]
              n168 = Concatenate Strings(w294, w293) -> (w292:string)
              n169 = Concatenate Strings(w292, w290, w291) -> (w284:string)
              n170 = local read "LKG Path"() -> (w286:path)
              n171 = Concatenate Strings(w285, w284) -> (w287:string)
              n172 = call <vilib>:"Write Characters To File.vi"("append to file? (new file:F)"=TRUE, "character string"=w287, "file path (dialog if empty)"=w286) -> ()  [unwired: 2 in, 1 out]
            }
          }
        }
      }
      n173 = call "HP415xA Sys-Error Query.vi"("VISA session"=w92, "error in (no error)"=w96) -> ("error out"=w118:errorcluster)  [unwired: 2 in, 1 out]
      n174 = call "HP415xA  Close.vi"("error in (no error)"=w118, "VISA session"=w92) -> ("error out"=w119:errorcluster)
      n175 = local write "error?"(w119) -> ()
    }
  }
